vi "all_of_one.vi"() -> ()   [LabVIEW 2020]
uses:
  c112fc2c-5164-4be4-9a52-92eec6d539c9.vi
  3d77a3c8-4017-4604-99a2-a5cb9d14e92c.vi
  <vilib>/Instr/_visa.llb/VISA Configure Serial Port (Instr).vi
  <vilib>/Utility/file.llb/Read Delimited Spreadsheet (DBL).vi
panel:
  out "stop":bool
  in  "Tab Control":enum32{"Path", "GPS", "LiDAR", "ETC"}(tab)
  out "CMD_2_ERP":T1
  out "Tracking_Error(m)":dbl
  in  "A/M":bool=TRUE
  in  "Vel":dbl=4.0 format="%#_13g"
  out "Index(near vehicle)":i32
  out "Steer_CMD(Deg)":dbl
  out "XY Graph 2":T2(graph)
  out "ERP_Receive":T3
  in  "file path (dialog if empty)":path caption="RDDF"
  out "TM_X(lat)":dbl format="%-#_10g M"
  out "TM_Y(long)":dbl format="%-#_10g M"
  in  "Serial Name":refnum<visa-resource-name>="COM8"
  out "ERP_Serial_DATA(RAW)":string
  out "Brake":u8
  out "XYGraph":cluster{"array":dbl[], "array":dbl[]}[](graph)
  in  "VISA resource name":refnum<visa-resource-name>
  in  "baud rate (115200)":u32=9600
  out "True Heading":string
  out "도분초(lon)":string
  out "도(lon)":string
  out "도분초(lat)":string
  out "도(lat)":string
  out "Latitude":dbl
  out "Longtitude":dbl
  out "UTC":dbl
  out "error out":errorcluster
  out "X(N)":dbl format="%#_6f"
  out "Y(E)":dbl format="%#_6f"
  in  "Refresh":bool
  out "WP_no.":i32
  out "Satellited Used":string
  out "Fix Position":string
  out "XY Graph":cluster{dbl[], dbl[]}(graph)
  out "Mixed Signal Graph":cluster{dbl[], dbl[]}[](graph)
  out "seconds":dbl
  out "minutes":dbl
  in  "channel 15":bool
  in  "channel 14":bool
  in  "channel 13":bool
  in  "channel 12":bool
  in  "channel 11":bool
  in  "channel 10":bool
  in  "channel 9":bool=TRUE
  in  "channel 8":bool=TRUE
  in  "channel 7":bool=TRUE
  in  "channel 6":bool=TRUE
  in  "channel 5":bool
  in  "channel 4":bool
  in  "channel 3":bool
  in  "channel 2":bool
  in  "channel 1":bool
  in  "channel 0":bool
  in  "range(m)":dbl
  in  "점 개수":i32
  out "Path_Vel_arr":dbl[](array[numeric])
  out "Path_long_arr":dbl[](array[numeric])
  out "Path_lat_arr":dbl[](array[numeric])
  out "x_lat_path":dbl[](array[numeric])
  out "y_long_path":dbl[](array[numeric])
  out "vel. path":dbl[](array[numeric])
  out "Heading_T":dbl
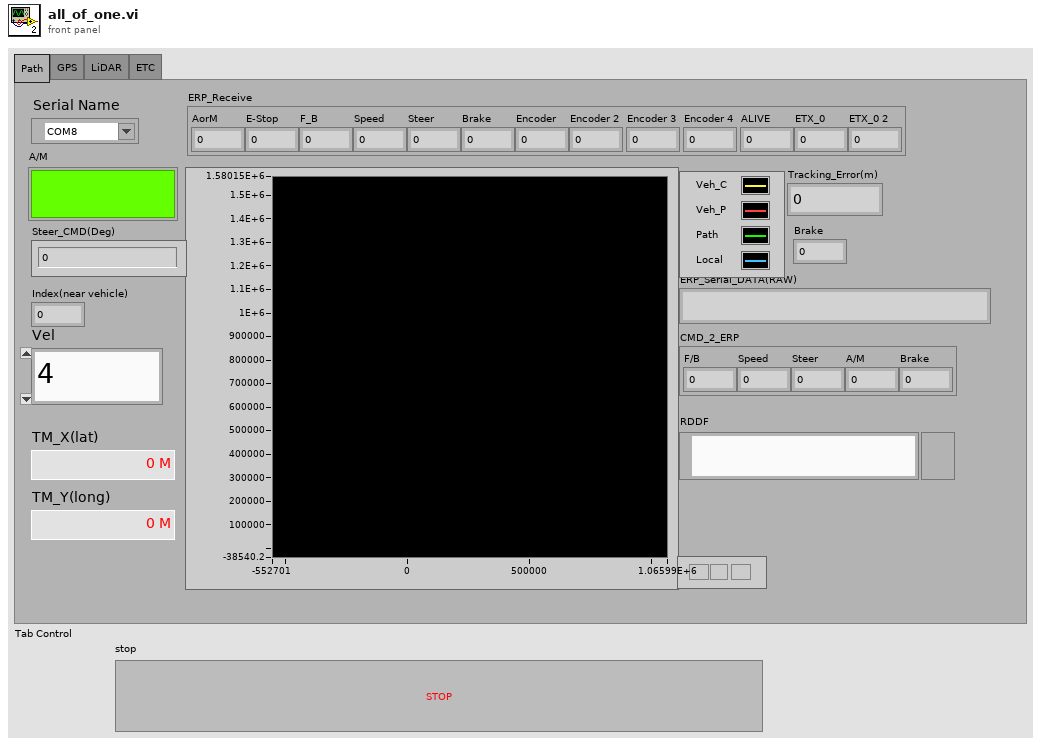
[diagram p1: front panel]
types:
  T1 = cluster{"F/B":u8, "Speed":u16, "Steer":i16, "A/M":u8, "Brake":u8}
  T2 = cluster{"y_long_path":dbl[], "x_lat_path":dbl[]}[]
  T3 = cluster{"AorM":u8, "E-Stop":u8, "F_B":u8, "Speed":u16, "Steer":i16, "Brake":u8, "Encoder":u8, "Encoder 2":u8, "Encoder 3":u8, "Encoder 4":u8, "ALIVE":u8, "ETX_0":u8, "ETX_0 2":u8}
  T4 = enum16{"open", "replace", "create", "open or create", "replace or create", "replace or create with confirmation"}
  T5 = cluster{"Path_long_arr":dbl[], "Path_lat_arr":dbl[]}
  T6 = cluster{"Path_long_arr":dbl[], "Path_lat_arr":dbl[]}[]
  T7 = cluster{"S":u8, "T":u8, "X":u8, "AorM":u8, "E-Stop":u8, "F_B":u8, "Speed":u16, "Steer":i16, "Brake":u8, "ALIVE":u8, "ETX_0":u8, "ETX_0 2":u8}
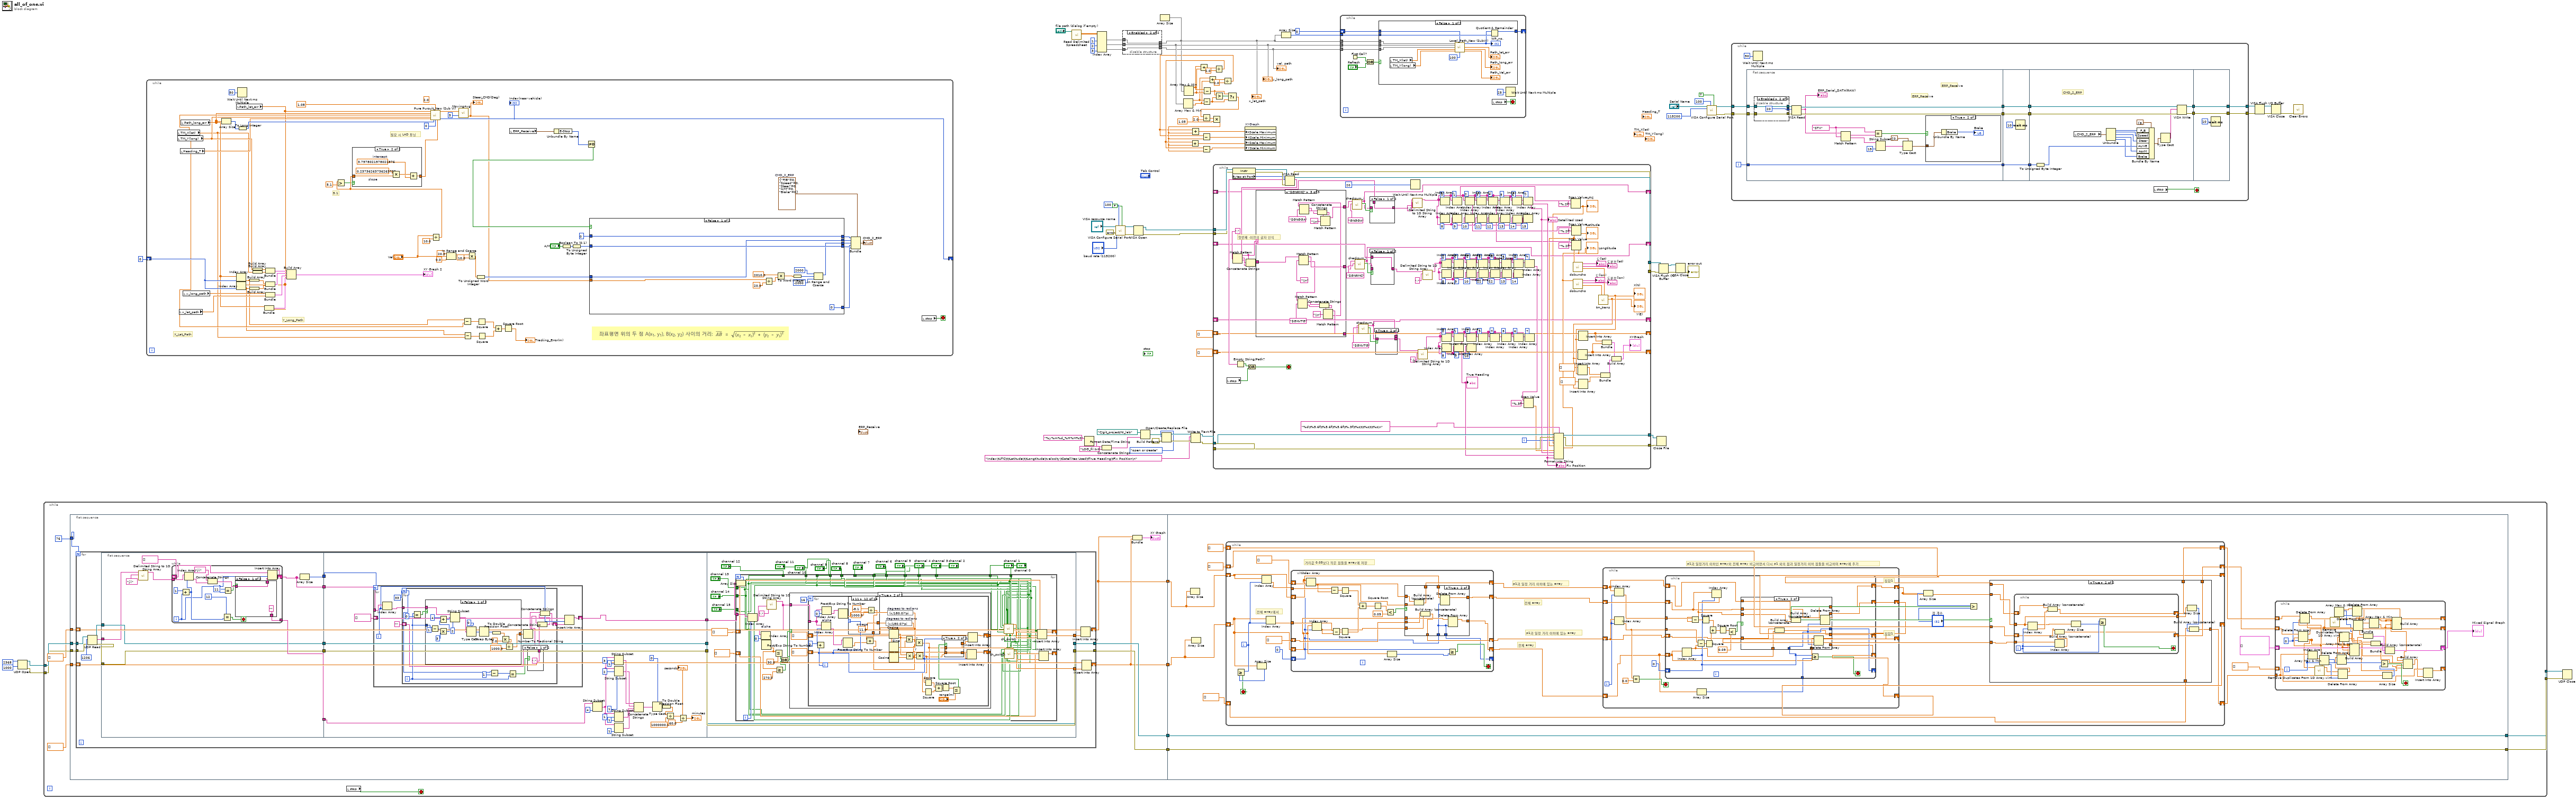
[diagram p0: block diagram]
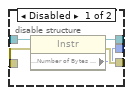
[diagram p2: hidden frame]
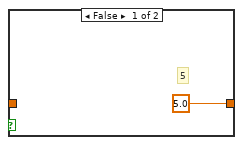
[diagram p4: hidden frame]
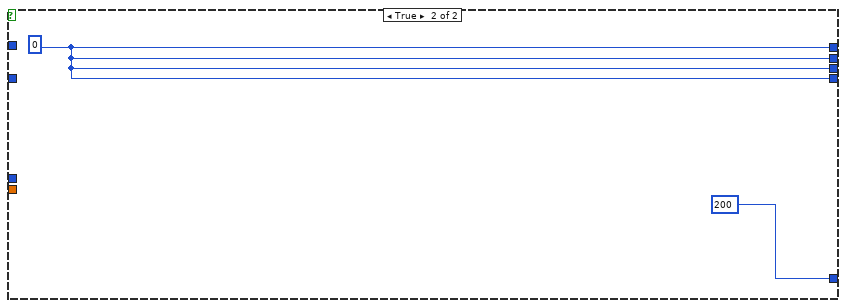
[diagram p5: hidden frame]
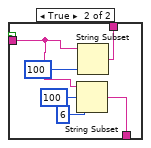
[diagram p6: hidden frame]
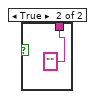
[diagram p7: hidden frame]
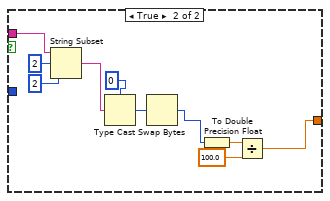
[diagram p8: hidden frame]
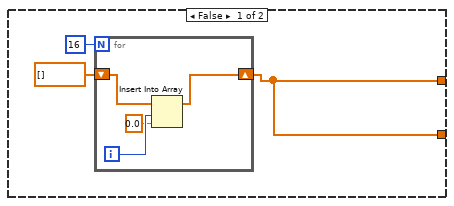
[diagram p9: hidden frame]
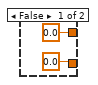
[diagram p10: hidden frame]
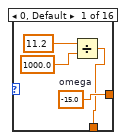
[diagram p11: hidden frame]
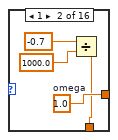
[diagram p12: hidden frame]
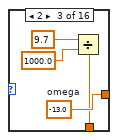
[diagram p13: hidden frame]
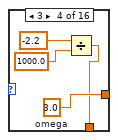
[diagram p14: hidden frame]
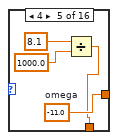
[diagram p15: hidden frame]
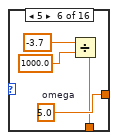
[diagram p16: hidden frame]
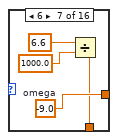
[diagram p17: hidden frame]
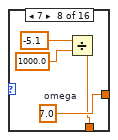
[diagram p18: hidden frame]
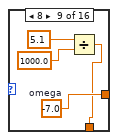
[diagram p19: hidden frame]
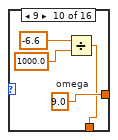
[diagram p20: hidden frame]
diagram:
  n1 = UDP Open(9:1000 ("timeout ms (25000)"), 11:u16 2368 ("port")) -> (port=w16:refnum<k16>, 0:w15:errorcluster)  [unwired: 3 in, 1 out]
  n2 = while {
    tunnel: w16 -> [w95]
    tunnel: w15 -> [w94]
    tunnel: [w91] -> w14
    tunnel: [w96] -> w13
    stop <- w85 stop-if-true
    n3 = flat-sequence {
      tunnel: w95 -> [w105]
      tunnel: w94 -> [w104]
      tunnel: dbl[] [] -> [w103]
      tunnel: dbl[] [] -> [w102]
      tunnel: 76 -> [w100]
      tunnel: [w106] -> w89
      tunnel: [w101] -> w88
      tunnel: [w98] -> w87
      tunnel: [w97] -> w86
      tunnel: [w427] -> w91
      tunnel: [w428] -> w96
      tunnel: w89 -> [w428]
      tunnel: w88 -> [w427]
      tunnel: w87 -> [w420]
      tunnel: w86 -> [w419]
      frame #0 {
        n4 = for {
          N: w100 -> [_]
          tunnel: w105 -> [w117]
          tunnel: [w119] -> w101
          tunnel: w104 -> [w116]
          tunnel: [w120] -> w106
          shift-right: [w109] -> w97
          shift-left: w103 -> [w108]
          shift-right: [w111] -> w98
          shift-left: w102 -> [w107]
          n5 = UDP Read(connection ID=w117, max size (548)=1206, 8:w116) -> (data out=w113:string, error out=w114:errorcluster, 3:w115:refnum<k16>)  [unwired: 1 in, 2 out]
          n6 = flat-sequence {
            tunnel: [w131] -> w128
            tunnel: [w130] -> w127
            tunnel: [w134] -> w126
            tunnel: [w133] -> w125
            tunnel: [w132] -> w124
            tunnel: w114 -> [w131]
            tunnel: w115 -> [w130]
            tunnel: w113 -> [w129]
            tunnel: w128 -> [w188]
            tunnel: w127 -> [w187]
            tunnel: w126 -> [w186]
            tunnel: w125 -> [w185]
            tunnel: w124 -> [w183]
            tunnel: [w188] -> w123
            tunnel: [w187] -> w122
            tunnel: [w161] -> w121
            tunnel: [w263] -> w119
            tunnel: [w264] -> w120
            tunnel: w123 -> [w264]
            tunnel: w122 -> [w263]
            tunnel: w121 -> [w261]
            tunnel: [w258] -> w110
            tunnel: [w257] -> w112
            frame #0 {
              n7 = call <vilib>:"Delimited String to 1D String Array.vi"("delimiter"="ÿî", "delimited string"=w129) -> ("string array"=w135:string[])  [unwired: 9 in]
              n8 = while {
                tunnel: w135 -> [w152]
                shift-right: [w145] -> w133
                shift-left: string[] [] -> [w144]
                tunnel: [w138] -> w132
                i -> [w141]
                stop <- w146 stop-if-true
                n9 = Add(x=1, y=w141) -> (x+y=w148:i32)
                n10 = Index Array(array=w152, index=w148) -> (element=w151:string)
                n11 = Concatenate Strings("ÿî" ("delimiter"), w151) -> (w143:string)
                n12 = Equal?(x=12, y=w148) -> (x = y?=w146:bool)
                n13 = Equal?(x=11, y=w141) -> (x = y?=w139:bool)
                n14 = case shown="False" w139 {
                  tunnel: w143 -> [w154 w156]
                  tunnel: [w154 w159] -> w142
                  tunnel: ["" w155] -> w138
                  frame False {
                  }
                  frame True {
                    n15 = String Subset(string=w156, offset (0)=100, length (rest)=6 ("length (rest)")) -> (substring=w155:string)
                    n16 = String Subset(string=w156, length (rest)=100 ("length (rest)")) -> (substring=w159:string)  [unwired: 1 in]
                  }
                }
                n17 = Insert Into Array(array=w144, index=w141, new element=w142) -> (w145:string[])
              }
              n18 = Array Size(array=w133) -> (size(s)=w134:i32)
            }
            frame #1 {
              n19 = for {
                N: w186 -> [_]
                tunnel: w185 -> [w196]
                shift-right: [w192] -> w161
                shift-left: string[] [] -> [w190]
                i -> [w193]
                n20 = Index Array(array=w196, index=w193) -> (element=w194:string)
                n21 = for {
                  N: 33 -> [w199]
                  tunnel: w194 -> [w208]
                  shift-right: [w201] -> w191
                  shift-left: "" -> [w200]
                  i -> [w207]
                  n22 = Equal?(x=w207, y=0) -> (x = y?=w209:bool)
                  n23 = case shown="False" w209 {
                    tunnel: w208 -> [w220 w238]
                    tunnel: w207 -> [w225 _]
                    tunnel: [w213 w231] -> w205
                    frame False {
                      n24 = Subtract(x=w225, y=1) -> (x-y=w226:i32)
                      n25 = Multiply(x=w226, y=3) -> (x*y=w222:i32)
                      n26 = Add(x=4 ("offset (0)"), y=w222) -> (x+y=w221:i32)
                      n27 = String Subset(string=w220, offset (0)=w221, length (rest)=2 ("length (rest)")) -> (substring=w219:string)
                      n28 = Type Cast(type=u16 0, x=w219) -> (*(type *) &x=w228:u16)
                      n29 = Swap Bytes(anything=w228) -> (byte swapped=w218:u16)
                      n30 = To Double Precision Float(number=w218) -> (double precision float=w217:dbl)
                      n31 = Multiply(x=w217, y=2.0) -> (x*y=w214:dbl)
                      n32 = Divide(x=w214, y=1000.0) -> (x/y=w213:dbl)
                    }
                    frame True {
                      n33 = String Subset(string=w238, offset (0)=2, length (rest)=2 ("length (rest)")) -> (substring=w235:string)
                      n34 = Type Cast(type=u16 0, x=w235) -> (*(type *) &x=w236:u16)
                      n35 = Swap Bytes(anything=w236) -> (byte swapped=w233:u16)
                      n36 = To Double Precision Float(number=w233) -> (double precision float=w234:dbl)
                      n37 = Divide(x=w234, y=100.0) -> (x/y=w231:dbl)
                    }
                  }
                  n38 = Subtract(x=w199, y=1) -> (x-y=w197:i32)
                  n39 = Equal?(x=w197, y=w207) -> (x = y?=w206:bool)
                  n40 = Number To Fractional String(number=w205) -> (F-format string=w204:string)  [unwired: 3 in]
                  n41 = case shown="False" w206 {
                    tunnel: ["," ""] -> w203
                    frame False {
                    }
                    frame True {
                    }
                  }
                  n42 = Concatenate Strings(w204, w203) -> (w202:string)
                  n43 = Concatenate Strings(w200, w202) -> (w201:string)
                }
                n44 = Insert Into Array(array=w190, index=w193, new element=w191) -> (w192:string[])
              }
              n45 = String Subset(string=w183, length (rest)=4 ("length (rest)")) -> (substring=w181:string)  [unwired: 1 in]
              n46 = String Subset(string=w181, offset (0)=3, length (rest)=1 ("length (rest)")) -> (substring=w173:string)
              n47 = String Subset(string=w181, offset (0)=2, length (rest)=1 ("length (rest)")) -> (substring=w172:string)
              n48 = String Subset(string=w181, offset (0)=1, length (rest)=1 ("length (rest)")) -> (substring=w171:string)
              n49 = String Subset(string=w181, length (rest)=1 ("length (rest)")) -> (substring=w170:string)  [unwired: 1 in]
              n50 = Concatenate Strings(w173, w172, w171, w170) -> (w168:string)
              n51 = Type Cast(type=u32 0, x=w168) -> (*(type *) &x=w167:u32)
              n52 = To Double Precision Float(number=w167) -> (double precision float=w166:dbl)
              n53 = Divide(x=w166, y=1000000.0) -> (x/y=w163:dbl)
              "seconds" <- w163
              n54 = Divide(x=w163, y=60.0) -> (x/y=→"minutes":dbl)
            }
            frame #2 {
              n55 = Array Size(array=w261) -> (size(s)=w262:i32)
              n56 = for {
                N: w262 -> [_]
                tunnel: w261 -> [w300]
                shift-right: [w297] -> w258
                shift-left: dbl[] [] -> [w296]
                shift-right: [w295] -> w257
                shift-left: dbl[] [] -> [w294]
                tunnel: "channel 0" -> [w289]
                tunnel: "channel 1" -> [w288]
                tunnel: "channel 2" -> [w287]
                tunnel: "channel 3" -> [w286]
                tunnel: "channel 4" -> [w285]
                tunnel: "channel 5" -> [w284]
                tunnel: "channel 6" -> [w283]
                tunnel: "channel 7" -> [w282]
                tunnel: "channel 8" -> [w281]
                tunnel: "channel 9" -> [w280]
                tunnel: "channel 10" -> [w279]
                tunnel: "channel 11" -> [w278]
                tunnel: "channel 12" -> [w277]
                tunnel: "channel 13" -> [w276]
                tunnel: "channel 14" -> [w275]
                tunnel: "channel 15" -> [w274]
                i -> [w298]
                n57 = Index Array(array=w300, index=w298) -> (element=w299:string)
                n58 = call <vilib>:"Delimited String to 1D String Array.vi"("delimiter"=",", "delimited string"=w299) -> ("string array"=w273:string[])  [unwired: 9 in]
                n59 = Index Array "alpha"(array=w273, index=0) -> (element=w271:string)
                n60 = Fract/Exp String To Number(string=w271) -> (number=w269:dbl)  [unwired: 3 in, 1 out]
                n61 = Less Or Equal?(x=w269, y=90.0 ("작거나같다")) -> (x <= y?=w267:bool)
                n62 = Greater Or Equal?(x=w269, y=270.0 ("크거나같다")) -> (x >= y?=w266:bool)
                n63 = Or(x=w267, y=w266) -> (x .or. y?=w265:bool)
                n64 = case shown="True" w265 {
                  tunnel: [w302 w311] -> w291
                  tunnel: [w302 w310] -> w290
                  tunnel: w273 -> [_ w309]
                  frame False {
                    n65 = for {
                      N: 16 -> [_]
                      shift-right: [w308] -> w302
                      shift-left: dbl[] [] -> [w305]
                      i -> [w307]
                      n66 = Insert Into Array(array=w305, index=w307, new element=0.0 ("new element/subarray")) -> (w308:dbl[])
                    }
                  }
                  frame True {
                    n67 = for {
                      N: 16 -> [_]
                      tunnel: w309 -> [w345]
                      shift-right: [w332] -> w311
                      shift-left: dbl[] [] -> [w331]
                      shift-right: [w329] -> w310
                      shift-left: dbl[] [] -> [w328]
                      i -> [w330]
                      n68 = Add(x=1, y=w330) -> (x+y=w346:i32)
                      n69 = Index Array(array=w345, index=w346) -> (element=w342:string)
                      n70 = Index Array "alpha"(array=w345, index=0) -> (element=w343:string)
                      n71 = Fract/Exp String To Number(string=w343) -> (number=w333:dbl)  [unwired: 3 in, 1 out]
                      n72 = Fract/Exp String To Number(string=w342) -> (number=w326:dbl)  [unwired: 3 in, 1 out]
                      n73 = case shown="11" w330 {
                        tunnel: [w355 w359 w363 w367 w371 w375 w379 w383 w387 w391 w395 w399 w403 w407 w411 w415] -> w341
                        tunnel: [w352 w356 w360 w364 w368 w372 w376 w380 w384 w388 w392 w396 w400 w404 w408 w412] -> w327
                        frame 0, Default {
                          w355 = -15.0  # omega
                          n74 = Divide(x=11.2, y=1000.0) -> (x/y=w352:dbl)
                        }
                        frame 1 {
                          w359 = 1.0  # omega
                          n75 = Divide(x=-0.7, y=1000.0) -> (x/y=w356:dbl)
                        }
                        frame 2 {
                          w363 = -13.0  # omega
                          n76 = Divide(x=9.7, y=1000.0) -> (x/y=w360:dbl)
                        }
                        frame 3 {
                          w367 = 3.0  # omega
                          n77 = Divide(x=-2.2, y=1000.0) -> (x/y=w364:dbl)
                        }
                        frame 4 {
                          w371 = -11.0  # omega
                          n78 = Divide(x=8.1, y=1000.0) -> (x/y=w368:dbl)
                        }
                        frame 5 {
                          w375 = 5.0  # omega
                          n79 = Divide(x=-3.7, y=1000.0) -> (x/y=w372:dbl)
                        }
                        frame 6 {
                          w379 = -9.0  # omega
                          n80 = Divide(x=6.6, y=1000.0) -> (x/y=w376:dbl)
                        }
                        frame 7 {
                          w383 = 7.0  # omega
                          n81 = Divide(x=-5.1, y=1000.0) -> (x/y=w380:dbl)
                        }
                        frame 8 {
                          w387 = -7.0  # omega
                          n82 = Divide(x=5.1, y=1000.0) -> (x/y=w384:dbl)
                        }
                        frame 9 {
                          w391 = 9.0  # omega
                          n83 = Divide(x=-6.6, y=1000.0) -> (x/y=w388:dbl)
                        }
                        frame 10 {
                          w395 = -5.0  # omega
                          n84 = Divide(x=3.7, y=1000.0) -> (x/y=w392:dbl)
                        }
                        frame 11 {
                          w399 = 11.0  # omega
                          n85 = Divide(x=-8.1, y=1000.0) -> (x/y=w396:dbl)
                        }
                        frame 12 {
                          w403 = -3.0  # omega
                          n86 = Divide(x=2.2, y=1000.0) -> (x/y=w400:dbl)
                        }
                        frame 13 {
                          w407 = 13.0  # omega
                          n87 = Divide(x=-9.7, y=1000.0) -> (x/y=w404:dbl)
                        }
                        frame 14 {
                          w411 = -1.0  # omega
                          n88 = Divide(x=0.7, y=1000.0) -> (x/y=w408:dbl)
                        }
                        frame 15 {
                          w415 = 15.0  # omega
                          n89 = Divide(x=-11.2, y=1000.0) -> (x/y=w412:dbl)
                        }
                      }
                      n90 = Add(x=w327, y=w326) -> (x+y=w325:dbl)
                      n91 = expression code="(x/180.0)*pi" "degrees to radians"(w341) -> (w340:dbl)
                      n92 = expression code="(x/180.0)*pi" "degrees to radians"(w333) -> (w339:dbl)
                      n93 = Cosine(x=w340) -> (cos(x)=w337:dbl)
                      n94 = Sine(x=w339) -> (sin(x)=w338:dbl)
                      n95 = Cosine(x=w339) -> (cos(x)=w336:dbl)
                      n96 = Multiply(x=w337, y=w338) -> (x*y=w334:dbl)
                      n97 = Multiply(x=w337, y=w336) -> (x*y=w335:dbl)
                      n98 = Multiply "x"(x=w334, y=w325) -> (x*y=w319:dbl)
                      n99 = Multiply "y"(x=w335, y=w325) -> (x*y=w317:dbl)
                      n100 = Square(x=w319) -> (x^2=w324:dbl)
                      n101 = Square(x=w317) -> (x^2=w323:dbl)
                      n102 = Add(x=w324, y=w323) -> (x+y=w322:dbl)
                      n103 = Square Root(x=w322) -> (sqrt(x)=w321:dbl)
                      n104 = Less Or Equal?(x=w321, y="range(m)") -> (x <= y?=w320:bool)
                      n105 = case shown="True" w320 {
                        tunnel: w319 -> [_ w351]
                        tunnel: [0.0 w351] -> w318
                        tunnel: w317 -> [_ w350]
                        tunnel: [0.0 w350] -> w316
                        frame False {
                        }
                        frame True {
                        }
                      }
                      n106 = Insert Into Array(array=w328, index=w330, new element=w316) -> (w329:dbl[])
                      n107 = Insert Into Array(array=w331, index=w330, new element=w318) -> (w332:dbl[])
                    }
                  }
                }
                n108 = call "ch_switch.vi"("channel 14"=w275, "channel 4"=w285, "channel 13"=w276, "channel 5"=w284, "channel 12"=w277, "channel 6"=w283, "channel 7"=w282, "channel 3"=w286, "channel 8"=w281, "channel 15"=w274, "channel 9"=w280, "channel 2"=w287, "channel 10"=w279, "channel 1"=w288, "channel 11"=w278, "channel 0"=w289, "Array in"=w291) -> ("Array out"=w292:dbl[])  [unwired: 10 in]
                n109 = call "ch_switch.vi"("channel 14"=w275, "channel 4"=w285, "channel 13"=w276, "channel 5"=w284, "channel 12"=w277, "channel 6"=w283, "channel 7"=w282, "channel 3"=w286, "channel 8"=w281, "channel 15"=w274, "channel 9"=w280, "channel 2"=w287, "channel 10"=w279, "channel 1"=w288, "channel 11"=w278, "channel 0"=w289, "Array in"=w290) -> ("Array out"=w293:dbl[])  [unwired: 10 in]
                n110 = Insert Into Array(array=w296, new element=w292) -> (w297:dbl[])  [unwired: 1 in]
                n111 = Insert Into Array(array=w294, new element=w293) -> (w295:dbl[])  [unwired: 1 in]
              }
            }
          }
          n112 = Insert Into Array(array=w108, new element=w110) -> (w109:dbl[])  [unwired: 1 in]
          n113 = Insert Into Array(array=w107, new element=w112) -> (w111:dbl[])  [unwired: 1 in]
        }
        n114 = Bundle(w97, w98) -> (→"XY Graph":cluster{dbl[], dbl[]})  [unwired: 1 in]
      }
      frame #1 {
        n115 = Array Size(array=w419) -> ()  [unwired: 1 out]
        n116 = Array Size(array=w420) -> ()  [unwired: 1 out]
        n117 = while {
          shift-right: [w471] -> _
          shift-left: w419 -> [w480]
          shift-right: [w475] -> _
          shift-left: w420 -> [w479]
          shift-right: [w472] -> w423
          shift-left: dbl[] [] -> [w474]
          shift-right: [w469] -> w422
          shift-left: dbl[] [] -> [w473]
          shift-right: [w467] -> w421
          shift-left: dbl[] [] -> [w468]
          i -> [w488]
          stop <- w489 stop-if-true
          # "전체 array에서"
          # "전체 array"
          # "p1과 일정 거리 이하에 있는 array"
          # "전체 array"
          # "p1과 일정거리 이하인 array와 전체 array 비교하면서 다시 p1 외의 점과 일정거리 이하 점들을 비교하며 array에 추가"
          # "p1과 일정 거리 이하에 있는 array"
          # "거리값 0.05보다 작은 점들을 array에 저장"
          n118 = Array Size(array=w479) -> (size(s)=w490:i32)
          n119 = Greater Or Equal?(x=w488, y=w490) -> (x >= y?=w489:bool)
          n120 = Index Array(array=w480, index=w488) -> (element=w487:dbl)
          n121 = Index Array(array=w479, index=w488) -> (element=w486:dbl)
          n122 = while {
            tunnel: w487 -> [w595]
            tunnel: w486 -> [w594]
            shift-right: [w580] -> w470
            shift-left: dbl[] [] ("array") -> [w582]
            shift-right: [w581] -> w466
            shift-left: dbl[] [] ("array") -> [w583]
            shift-right: [w577] -> w465
            shift-left: w480 -> [w579]
            shift-right: [w576] -> w464
            shift-left: w479 -> [w578]
            shift-right: [w572] -> _
            shift-left: 0 -> [w573]
            stop <- w574 stop-if-true
            n123 = Index Array(array=w579, index=w573) -> (element=w585:dbl)
            n124 = Index Array(array=w578, index=w573) -> (element=w584:dbl)
            n125 = Subtract(x=w595, y=w585) -> (x-y=w593:dbl)
            n126 = Subtract(x=w594, y=w584) -> (x-y=w592:dbl)
            n127 = Square(x=w592) -> (x^2=w590:dbl)
            n128 = Square(x=w593) -> (x^2=w591:dbl)
            n129 = Add(x=w591, y=w590) -> (x+y=w589:dbl)
            n130 = Square Root(x=w589) -> (sqrt(x)=w588:dbl)
            n131 = Less?(x=w588, y=0.09) -> (x < y?=w586:bool)
            n132 = Array Size(array=w578) -> (size(s)=w575:i32)
            n133 = case shown="True" w586 {
              tunnel: w583 -> [w602 w610]
              tunnel: w582 -> [w601 w607]
              tunnel: w585 -> [_ w609]
              tunnel: w584 -> [_ w606]
              tunnel: [w602 w608] -> w581
              tunnel: [w601 w605] -> w580
              tunnel: w579 -> [w600 w613]
              tunnel: [w600 w604] -> w577
              tunnel: w578 -> [w599 w612]
              tunnel: [w599 w611] -> w576
              tunnel: w573 -> [w597 w603]
              tunnel: [w596 w603] -> w572
              frame False {
                n134 = Add(x=1, y=w597) -> (x+y=w596:i32)
              }
              frame True {
                n135 = Build Array (concatenate)(w610, w609) -> (w608:dbl[])
                n136 = Build Array (concatenate)(w607, w606) -> (w605:dbl[])
                n137 = Delete From Array(array=w613, index=w603) -> (array with subset deleted=w604:dbl[])  [unwired: 1 in, 1 out]
                n138 = Delete From Array(array=w612, index=w603) -> (array with subset deleted=w611:dbl[])  [unwired: 1 in, 1 out]
              }
            }
            n139 = Greater Or Equal?(x=w573, y=w575) -> (x >= y?=w574:bool)
          }
          n140 = while {
            shift-right: [w521] -> w477
            shift-left: w466 -> [w524]
            shift-right: [w527] -> w476
            shift-left: w470 -> [w526]
            shift-right: [w522] -> w471
            shift-left: w465 -> [w525]
            shift-right: [w528] -> w475
            shift-left: w464 -> [w515]
            i -> [w520]
            stop <- w517 stop-if-true
            # "집합1"
            # "집합1"
            n141 = Index Array(array=w526, index=w520) -> (element=w518:dbl)
            n142 = Index Array(array=w524, index=w520) -> (element=w523:dbl)
            n143 = Equal?(x=w518, y=0.0) -> (x = y?=w517:bool)
            n144 = Array Size(array=w515) -> (size(s)=w516:i32)
            n145 = while {
              tunnel: w523 -> [w553]
              tunnel: w518 -> [w552]
              shift-right: [w540] -> _
              shift-left: 0 -> [w541]
              shift-right: [w536] -> w527
              shift-left: w526 -> [w533]
              shift-right: [w532] -> w521
              shift-left: w524 -> [w539]
              shift-right: [w531] -> w522
              shift-left: w525 -> [w535]
              shift-right: [w538] -> w528
              shift-left: w515 -> [w537]
              tunnel: w516 -> [w530]
              stop <- w542 stop-if-true
              n146 = Index Array(array=w537, index=w541) -> (element=w534:dbl)
              n147 = Subtract(x=w552, y=w534) -> (x-y=w550:dbl)
              n148 = Square(x=w550) -> (x^2=w549:dbl)
              n149 = Index Array(array=w535, index=w541) -> (element=w543:dbl)
              n150 = Subtract(x=w553, y=w543) -> (x-y=w551:dbl)
              n151 = Square(x=w551) -> (x^2=w548:dbl)
              n152 = Add(x=w548, y=w549) -> (x+y=w547:dbl)
              n153 = Square Root(x=w547) -> (sqrt(x)=w546:dbl)
              n154 = Less?(x=w546, y=0.09) -> (x < y?=w544:bool)
              n155 = case shown="True" w544 {
                tunnel: w535 -> [w554 w563]
                tunnel: w541 -> [w559 w568]
                tunnel: w543 -> [_ w571]
                tunnel: [w555 w561] -> w532
                tunnel: w533 -> [w557 w570]
                tunnel: w539 -> [w555 w564]
                tunnel: w537 -> [w560 w569]
                tunnel: [w554 w565] -> w531
                tunnel: [w560 w566] -> w538
                tunnel: [w558 w568] -> w540
                tunnel: [w557 w567] -> w536
                tunnel: w534 -> [_ w562]
                frame False {
                  n156 = Add(x=1, y=w559) -> (x+y=w558:i32)
                }
                frame True {
                  n157 = Build Array (concatenate)(w570, w562) -> (w567:dbl[])
                  n158 = Build Array (concatenate)(w564, w571) -> (w561:dbl[])
                  n159 = Delete From Array(array=w569, index=w568) -> (array with subset deleted=w566:dbl[])  [unwired: 1 in, 1 out]
                  n160 = Delete From Array(array=w563, index=w568) -> (array with subset deleted=w565:dbl[])  [unwired: 1 in, 1 out]
                }
              }
              n161 = Greater Or Equal?(x=w541, y=w530) -> (x >= y?=w542:bool)
            }
          }
          n162 = Array Size(array=w477) -> (size(s)=w482:i32)
          n163 = Greater?(x=w482, y="점 개수") -> (0:w483:bool)
          n164 = case shown="True" w483 {
            tunnel: w477 -> [_ w503]
            tunnel: w476 -> [_ w502]
            tunnel: w474 -> [w493 w501]
            tunnel: w473 -> [w492 w500]
            tunnel: [w493 w497] -> w472
            tunnel: [w492 w499] -> w469
            tunnel: w468 -> [w491 w496]
            tunnel: [w491 w495] -> w467
            frame False {
            }
            frame True {
              n165 = while {
                shift-right: [w506] -> w497
                shift-left: w501 -> [w509]
                tunnel: w503 -> [w504]
                shift-right: [w505] -> w499
                shift-left: w500 -> [w508]
                tunnel: w502 -> [w514]
                tunnel: [w504] -> w494
                i -> [w513]
                stop <- w511 stop-if-true
                n166 = Index Array(array=w504, index=w513) -> (element=w510:dbl)
                n167 = Build Array (concatenate)(w509, w510) -> (w506:dbl[])
                n168 = Index Array(array=w514, index=w513) -> (element=w507:dbl)
                n169 = Build Array (concatenate)(w508, w507) -> (w505:dbl[])
                n170 = Array Size(array=w504) -> (size(s)=w512:i32)
                n171 = Greater Or Equal?(x=w513, y=w512) -> (x >= y?=w511:bool)
              }
              n172 = Array Size(array=w494) -> (size(s)=w498:i32)
              n173 = Build Array (concatenate)(w496, w498) -> (w495:dbl[])
            }
          }
        }
        n174 = while {
          shift-right: [w458] -> _
          shift-left: w423 -> [w463]
          shift-right: [w455] -> _
          shift-left: w422 -> [w456]
          tunnel: w421 -> [w459]
          shift-right: [w453] -> w416
          shift-left: cluster{dbl[], dbl[]}[] [] -> [w452]
          shift-right: [w429] -> _
          shift-left: dbl[] [] ("array") -> [w431]
          i -> [w460]
          stop <- w461 stop-if-true
          w451 = 0 ("index")
          n175 = Index Array(array=w459, index=w460) -> (element=w457:dbl)
          n176 = Delete From Array(array=w456, length=w457, index=w451) -> (deleted portion=w442:dbl[], array with subset deleted=w455:dbl[])
          n177 = Delete From Array(array=w463, length=w457, index=w451) -> (deleted portion=w448:dbl[], array with subset deleted=w458:dbl[])
          n178 = call "Remove Duplicates From 1D Array.vim"("array"=w442) -> ("array with duplicates removed"=w440:dbl[])  [unwired: 10 in]
          n179 = Array Max & Min(array=w440) -> (max index (indices)=w438:i32, min index (indices)=w441:i32)  [unwired: 2 out]
          n180 = call "Remove Duplicates From 1D Array.vim"("array"=w448) -> ("array with duplicates removed"=w446:dbl[])  [unwired: 10 in]
          n181 = Array Max & Min(array=w446) -> (max index (indices)=w445:i32, min index (indices)=w447:i32)  [unwired: 2 out]
          n182 = Delete From Array(array=w440, index=w441) -> (array with subset deleted=w439:dbl[])  [unwired: 1 in, 1 out]
          n183 = Delete From Array(array=w439, index=w438) -> (array with subset deleted=w437:dbl[])  [unwired: 1 in, 1 out]
          n184 = Array Max & Min(array=w437) -> (max value=w433:dbl, min value=w432:dbl)  [unwired: 2 out]
          n185 = Build Array(w433, w432, w432, w433, w433) -> (w450:dbl[])
          n186 = Delete From Array(array=w446, index=w447) -> (array with subset deleted=w444:dbl[])  [unwired: 1 in, 1 out]
          n187 = Delete From Array(array=w444, index=w445) -> (array with subset deleted=w443:dbl[])  [unwired: 1 in, 1 out]
          n188 = Array Max & Min(array=w443) -> (max value=w435:dbl, min value=w434:dbl)  [unwired: 2 out]
          n189 = Bundle(w448, w442) -> (w454:cluster{dbl[], dbl[]})  [unwired: 1 in]
          n190 = Array Size(array=w459) -> (size(s)=w462:i32)
          n191 = Greater?(x=w460, y=w462) -> (0:w461:bool)
          n192 = Build Array(w435, w435, w434, w434, w435) -> (w449:dbl[])
          n193 = Bundle(w449, w450) -> (w436:cluster{dbl[], dbl[]})  [unwired: 1 in]
          n194 = Build Array (concatenate)(w452, w454, w436) -> (w453:cluster{dbl[], dbl[]}[])
          n195 = Build Array(w435, w434, w433, w432) -> (w430:dbl[])
          n196 = Insert Into Array(array=w431, new element=w430) -> (w429:dbl[])  [unwired: 1 in]
        }
        "Mixed Signal Graph" <- w416
      }
    }
    n197 = local read "stop"() -> (w85:bool)
  }
  n198 = while {
    shift-right: [w661] -> _
    shift-left: 0 -> [w658]
    stop <- w667 stop-if-true
    w633 = T1 {"F/B"=0, "Speed"=0, "Steer"=0, "A/M"=0, "Brake"=0}  # CMD_2_ERP
    (unwired) 2.0 ("L")
    # "5.1"
    # "X_Lat_Path"
    # "Y_Long_Path"
    # "필요 시 LAD 튜닝"
    n199 = local read "TM_X(lat)"() -> (w627:dbl)
    n200 = local read "TM_Y(long)"() -> (w628:dbl)
    n201 = local read "x_lat_path"() -> (w637:dbl[])
    n202 = local read "Heading_T"() -> (w654:dbl)
    n203 = local read "Path_long_arr"() -> (w630:dbl[])
    n204 = local read "y_long_path"() -> (w638:dbl[])
    n205 = Array Size(array=w630) -> (size(s)=w662:i32)
    n206 = local read "Path_lat_arr"() -> (w629:dbl[])
    n207 = Index Array(array=w630, index=w658) -> (element=w618:dbl)
    n208 = Index Array(array=w629, index=w658) -> (element=w617:dbl)
    n209 = Wait Until Next ms Multiple(millisecond multiple=u32 50 ("ms 배수")) -> ()  [unwired: 1 out]
    n210 = To Long Integer(number=w662) -> (32bit integer=w660:i32)
    n211 = Build Array(w618) -> (w669:dbl[])
    n212 = Build Array(w617) -> (w668:dbl[])
    n213 = Build Array(w628) -> (w671:dbl[])
    n214 = Build Array(w627) -> (w670:dbl[])
    n215 = Bundle("Path_long_arr"=w630, "Path_lat_arr"=w629) -> (w650:T5)  [unwired: 1 in]
    n216 = Bundle(w671, w670) -> (w656:cluster{dbl[], dbl[]})  [unwired: 1 in]
    n217 = Bundle(w669, w668) -> (w655:cluster{dbl[], dbl[]})  [unwired: 1 in]
    n218 = Bundle("y_long_path"=w638, "x_lat_path"=w637) -> (w657:cluster{"y_long_path":dbl[], "x_lat_path":dbl[]})  [unwired: 1 in]
    n219 = Build Array(w656, w655, w657, w650) -> (→"XY Graph 2":T6)
    n220 = Divide(x="Vel", y=10.0) -> (x/y=w651:dbl)
    n221 = Greater?(x=w651, y=5.1) -> (0:w616:bool)
    n222 = case shown="True" w616 {
      tunnel: w651 -> [_ w677]
      tunnel: [5.0 w676] -> w653
      frame False {
        # "5"
      }
      frame True {
        w678 = 3.7978021978021976  # intercept
        w680 = 0.23736263736263735  # slope
        n223 = Multiply(x=w680, y=w677) -> (x*y=w679:dbl)
        n224 = Add(x=w679, y=w678) -> (x+y=w676:dbl)
      }
    }
    n225 = call "Pure Pursuit_New (Sub VI).vi"("x_lat_path"=w629, "L"=1.08, "y_long_path"=w630, "X_Current"=w627, "Y_Current"=w628, "Heading_Current"=w654, "#pnt"=w660, "WP no_pre"=0, "LAD"=w653) -> ("Steer_CMD(Deg)"=w626:dbl, "Index(near vehicle)"=w661:i32)  [unwired: 5 in]
    "Index(near vehicle)" <- w661
    n226 = In Range and Coerce(upper limit=20.0 ("상위 리미트"), x="Vel", lower limit=0.0 ("하위 리미트")) -> (coerced(x)=w642:dbl)  [unwired: 1 out]
    n227 = call "MovingAvg.vi"("입력"=w626, "이동평균을 구할 자료의 개수"=u16 5) -> ("이동평균"=w614:dbl)  [unwired: 2 out]
    "Steer_CMD(Deg)" <- w614
    n228 = Subtract(x=w618, y=w628) -> (x-y=w623:dbl)
    n229 = Subtract(x=w617, y=w627) -> (x-y=w622:dbl)
    n230 = Multiply(x=w642, y=10.0) -> (x*y=w640:dbl)
    n231 = To Unsigned Word Integer(number=w640) -> (unsigned 16bit integer=w646:u16)
    n232 = Square(x=w623) -> (x^2=w621:dbl)
    n233 = Square(x=w622) -> (x^2=w620:dbl)
    n234 = Add(x=w621, y=w620) -> (x+y=w619:dbl)
    n235 = Square Root(x=w619) -> (sqrt(x)=→"Tracking_Error(m)":dbl)
    n236 = local read "ERP_Receive"() -> (w664:T3)
    n237 = Unbundle By Name(w664) -> ("E-Stop"=w665:u8)
    n238 = Boolean To (0,1)(Boolean="A/M") -> (0, 1=w649:i16)
    n239 = To Unsigned Byte Integer(number=w649) -> (unsigned 8bit integer=w631:u8)
    n240 = Not Equal To 0?(x=w665) -> (x != 0?=w645:bool)
    n241 = case shown="False" w645 {
      tunnel: u8 0 -> [w693 _]
      tunnel: [w693 w695] -> w674
      tunnel: [w690 w695] -> w673
      tunnel: [w682 w695] -> w672
      tunnel: [w692 w695] -> w648
      tunnel: w631 -> [w692 _]
      tunnel: w614 -> [w691 _]
      tunnel: w646 -> [w690 _]
      tunnel: [u8 0 u8 200] -> w634
      frame False {
        n242 = Divide(x=w691, y=20.0) -> (x/y=w688:dbl)
        n243 = Multiply(x=2010.0, y=w688) -> (x*y=w687:dbl)
        n244 = To Word Integer(number=w687) -> (16bit integer=w689:i16)
        n245 = In Range and Coerce(upper limit=i16 2000 ("상위 리미트"), x=w689, lower limit=i16 -2000 ("하위 리미트")) -> (coerced(x)=w682:i16)  [unwired: 1 out]
      }
      frame True {
        w695 = u8 0
      }
    }
    n246 = Bundle(cluster=w633, "F/B"=w674, "Speed"=w673, "Steer"=w672, "A/M"=w648, "Brake"=w634) -> (→"CMD_2_ERP":T1)
    n247 = local read "stop"() -> (w667:bool)
  }
  n248 = call-poly <vilib>:"Read Delimited Spreadsheet.vi"("file path (dialog if empty)"="file path (dialog if empty)") -> ("all rows"=w23:dbl[][])  [unwired: 9 in, 5 out]
  n249 = Format Date/Time String(time format string (%c)="%y%m%d_%H%M%S") -> (date/time string=w56:string)  [unwired: 2 in]
  n250 = Index Array(array=w23, index (col) #1=1 ("비활성화된 인덱스 (열)"), index (col) #2=2 ("인덱스 (열)"), index (col) #3=3 ("인덱스 (열)")) -> (element #1=w50:dbl[], element #2=w49:dbl[], element #3=w48:dbl[])  [unwired: 3 in]
  n251 = Concatenate Strings(w56, "LOG_fil.txt" ("string")) -> (w54:string)
  n252 = call-poly "VISA Configure Serial Port"("VISA resource name"="VISA resource name", "timeout (10sec)"=u32 100, "Enable Termination\nChar (T)"=FALSE ("Enable Termination\nChar (T)"), "baud rate (9600)"="baud rate (115200)", "error in (no error)"=errorcluster {"status"=FALSE, "code"=0, "source"=""}) -> ("VISA resource name out"=w68:refnum<visa-resource-name>, "error out"=w69:errorcluster)  [unwired: 9 in]
  n253 = disable-structure shown="Enabled" {
    disable-tunnel: w50 -> [w702 w705]
    disable-tunnel: w49 -> [w701 w704]
    disable-tunnel: w48 -> [w700 w703]
    disable-tunnel: [w699 w704] -> w27
    disable-tunnel: [w698 w703] -> w25
    disable-tunnel: [w697 w705] -> w24
    frame Disabled {
      n254 = call "InfPath(SubVI).vi"("Mod dist."=20.0, "vel."=w700, "y_long"=w701, "x_lat"=w702) -> ("vel. path"=w698:dbl[], "y_long_path"=w699:dbl[], "x_lat_path"=w697:dbl[])  [unwired: 1 out]
    }
    frame Enabled {
    }
  }
  "x_lat_path" <- w24
  "y_long_path" <- w27
  "vel. path" <- w25
  n255 = VISA Open(error in (no error)=w69, VISA resource name=w68) -> (VISA resource name=w67:refnum<visa-resource-name>, error out=w66:errorcluster)  [unwired: 3 in]
  n256 = Build Path(base path=path "C:/git_project/NI_lab", name or relative path=w54) -> (appended path=w82:path)
  n257 = Array Size(array=w24) -> ()  [unwired: 1 out]
  n258 = Open/Create/Replace File(file path (use dialog)=w82, error in=errorcluster {"status"=FALSE, "code"=0, "source"=""}, operation (0:open)=T4."open or create") -> (refnum out=w83:refnum<file>, error out=w84:errorcluster)  [unwired: 3 in, 1 out]
  n259 = Array Max & Min(array=w27) -> (max value=w36:dbl, min value=w35:dbl)  [unwired: 2 out]
  n260 = Array Max & Min(array=w24) -> (max value=w42:dbl, min value=w41:dbl)  [unwired: 2 out]
  n261 = Write to Text File(file (use dialog)=w83, text="Index\tUTC\t\tLatitude\t\tLongtitude\tvelocity\tSatellites Used\tTrue Heading\tFix Position\n", error in=w84) -> (refnum out=w75:refnum<file>, error out=w74:errorcluster)  [unwired: 1 in, 1 out]
  n262 = Add(x=w42, y=w41) -> (x+y=w39:dbl)
  n263 = Subtract(x=w36, y=w35) -> (x-y=w45:dbl)
  n264 = Subtract(x=w42, y=w41) -> (x-y=w46:dbl)
  n265 = Add(x=w36, y=w35) -> (x+y=w38:dbl)
  n266 = while {
    tunnel: w74 -> [w776]
    tunnel: [w775] -> w76
    tunnel: w75 -> [w778]
    tunnel: [w777] -> w77
    tunnel: w67 -> [w773]
    tunnel: w66 -> [w772]
    tunnel: [w761] -> w65
    tunnel: [w760] -> w64
    shift-right: [w716] -> _
    shift-left: _ -> [w740]
    shift-right: [w712] -> _
    shift-left: _ -> [w738]
    shift-right: [w709] -> _
    shift-left: _ -> [w736]
    shift-right: [w734] -> _
    shift-left: dbl[] [] -> [w735]
    shift-right: [w732] -> _
    shift-left: dbl[] [] -> [w733]
    i -> [w759]
    stop <- w826 stop-if-true
    # "첫번째 ,이전의 글자 인식"
    n267 = local read "stop"() -> (w706:bool)
    n268 = property class="Instr"(reference=w773, error in=w772) -> (reference out=w771:refnum<visa-resource-name>, error out=w770:errorcluster, "Bytes at Port"=w758:u32)
    n269 = VISA Read(VISA resource name=w771, byte count=w758, error in (no error)=w770) -> (VISA resource name out=w761:refnum<visa-resource-name>, read buffer=w753:string, error out=w760:errorcluster)  [unwired: 1 out]
    n270 = Match Pattern(string=w753, regular expression=",") -> (before substring=w750:string, match substring=w749:string, after substring=w748:string)  [unwired: 1 in, 1 out]
    n271 = Empty String/Path?(string/path=w753) -> (empty?=w827:bool)
    n272 = Concatenate Strings(w750, w749, w748) -> (w751:string)
    n273 = Or(x=w827, y=w706) -> (x .or. y?=w826:bool)
    n274 = case shown="\"$GNRMC\"" w750 {
      tunnel: w751 -> [w850 w867 w882]
      tunnel: [w849 w859 w869] -> w718
      tunnel: [w842 w852 w881] -> w714
      tunnel: [w835 w865 w875] -> w710
      frame "$GNGGA", Default {
        n275 = Match Pattern(string=w850, regular expression="\\n") -> (before substring=w849:string, after substring=w848:string)  [unwired: 1 in, 2 out]
        n276 = Match Pattern(string=w848, regular expression="$GNRMC") -> (match substring=w845:string, after substring=w844:string)  [unwired: 1 in, 2 out]
        n277 = Concatenate Strings(w845, w844) -> (w843:string)
        n278 = Match Pattern(string=w843, regular expression="\\n") -> (before substring=w842:string, after substring=w839:string)  [unwired: 1 in, 2 out]
        n279 = Match Pattern(string=w839, regular expression="$GNVTG") -> (match substring=w837:string, after substring=w836:string)  [unwired: 1 in, 2 out]
        n280 = Concatenate Strings(w837, w836) -> (w840:string)
        n281 = Match Pattern(string=w840, regular expression="\\n") -> (before substring=w835:string)  [unwired: 1 in, 3 out]
      }
      frame "$GNVTG" {
        n282 = Match Pattern(string=w867, regular expression="\\n") -> (before substring=w865:string, after substring=w864:string)  [unwired: 1 in, 2 out]
        n283 = Match Pattern(string=w864, regular expression="$GNGGA") -> (match substring=w861:string, after substring=w860:string)  [unwired: 1 in, 2 out]
        n284 = Concatenate Strings(w861, w860) -> (w862:string)
        n285 = Match Pattern(string=w862, regular expression="\\n") -> (before substring=w859:string, after substring=w858:string)  [unwired: 1 in, 2 out]
        n286 = Match Pattern(string=w858, regular expression="$GNRMC") -> (match substring=w854:string, after substring=w853:string)  [unwired: 1 in, 2 out]
        n287 = Concatenate Strings(w854, w853) -> (w855:string)
        n288 = Match Pattern(string=w855, regular expression="\\n") -> (before substring=w852:string)  [unwired: 1 in, 3 out]
      }
      frame "$GNRMC" {
        n289 = Match Pattern(string=w882, regular expression="\\n") -> (before substring=w881:string, after substring=w880:string)  [unwired: 1 in, 2 out]
        n290 = Match Pattern(string=w880, regular expression="$GNVTG") -> (match substring=w876:string, after substring=w877:string)  [unwired: 1 in, 2 out]
        n291 = Concatenate Strings(w876, w877) -> (w878:string)
        n292 = Match Pattern(string=w878, regular expression="\\n") -> (before substring=w875:string, after substring=w874:string)  [unwired: 1 in, 2 out]
        n293 = Match Pattern(string=w874, regular expression="$GNGGA") -> (match substring=w871:string, after substring=w870:string)  [unwired: 1 in, 2 out]
        n294 = Concatenate Strings(w871, w870) -> (w872:string)
        n295 = Match Pattern(string=w872, regular expression="\\n") -> (before substring=w869:string)  [unwired: 1 in, 3 out]
      }
    }
    n296 = call "checksum_i.vi"("check dataName"="GNGGA", "string"=w718) -> ("Boolean"=w717:bool, "String"=w716:string)  [unwired: 8 in]
    n297 = call "checksum_i.vi"("check dataName"="$GNRMC", "string"=w714) -> ("Boolean"=w713:bool, "String"=w712:string)  [unwired: 8 in]
    n298 = call "checksum_i.vi"("check dataName"="$GNVTG", "string"=w710) -> ("Boolean"=w708:bool, "String"=w709:string)  [unwired: 8 in]
    n299 = case shown="False" w717 {
      tunnel: [w833 w834] -> w741
      tunnel: w716 -> [_ w834]
      tunnel: w740 -> [w833 _]
      frame False {
      }
      frame True {
      }
    }
    n300 = case shown="False" w713 {
      tunnel: w712 -> [_ w832]
      tunnel: [w831 w832] -> w739
      tunnel: w738 -> [w831 _]
      frame False {
      }
      frame True {
      }
    }
    n301 = case shown="True" w708 {
      tunnel: w709 -> [_ w830]
      tunnel: [w829 w830] -> w737
      tunnel: w736 -> [w829 _]
      frame False {
      }
      frame True {
      }
    }
    n302 = Wait Until Next ms Multiple(millisecond multiple=u32 20) -> ()  [unwired: 1 out]
    n303 = call <vilib>:"Delimited String to 1D String Array.vi"("delimiter"=",", "delimited string"=w741) -> ("string array"=w825:string[])  [unwired: 9 in]
    n304 = call <vilib>:"Delimited String to 1D String Array.vi"("delimiter"=",", "delimited string"=w737) -> ("string array"=w790:string[])  [unwired: 9 in]
    n305 = call <vilib>:"Delimited String to 1D String Array.vi"("delimiter"=",", "delimited string"=w739) -> ("string array"=w807:string[])  [unwired: 9 in]
    n306 = Index Array(array=w825, index=0) -> ()  [unwired: 1 out]
    n307 = Index Array(array=w825, index=8) -> ()  [unwired: 1 out]
    n308 = Index Array(array=w807, index=0) -> ()  [unwired: 1 out]
    n309 = Index Array(array=w790, index=0) -> ()  [unwired: 1 out]
    n310 = Index Array(array=w807, index=8) -> ()  [unwired: 1 out]
    n311 = Index Array(array=w790, index=8) -> ()  [unwired: 1 out]
    n312 = Index Array(array=w825, index=1) -> (element=w766:string)
    n313 = Index Array(array=w825, index=9) -> ()  [unwired: 1 out]
    n314 = Index Array(array=w807, index=1) -> ()  [unwired: 1 out]
    n315 = Index Array(array=w807, index=9) -> ()  [unwired: 1 out]
    n316 = Index Array(array=w790, index=1) -> (element=w769:string)
    "True Heading" <- w769
    n317 = Index Array(array=w790, index=9) -> ()  [unwired: 1 out]
    n318 = Index Array(array=w825, index=2) -> (element=w763:string)
    n319 = Index Array(array=w825, index=10) -> ()  [unwired: 1 out]
    n320 = Index Array(array=w807, index=2) -> ()  [unwired: 1 out]
    n321 = Index Array(array=w807, index=10) -> ()  [unwired: 1 out]
    n322 = Index Array(array=w790, index=2) -> ()  [unwired: 1 out]
    n323 = Index Array(array=w790, index=10) -> ()  [unwired: 1 out]
    n324 = Index Array(array=w825, index=3) -> ()  [unwired: 1 out]
    n325 = Index Array(array=w825, index=11) -> ()  [unwired: 1 out]
    n326 = Index Array(array=w807, index=3) -> ()  [unwired: 1 out]
    n327 = Index Array(array=w790, index=3) -> ()  [unwired: 1 out]
    n328 = Index Array(array=w807, index=11) -> ()  [unwired: 1 out]
    n329 = Index Array(array=w825, index=4) -> (element=w762:string)
    n330 = Index Array(array=w825, index=12) -> ()  [unwired: 1 out]
    n331 = Index Array(array=w807, index=4) -> ()  [unwired: 1 out]
    n332 = Index Array(array=w790, index=4) -> ()  [unwired: 1 out]
    n333 = Index Array(array=w807, index=12) -> ()  [unwired: 1 out]
    n334 = Index Array(array=w825, index=5) -> ()  [unwired: 1 out]
    n335 = Index Array(array=w825, index=13) -> ()  [unwired: 1 out]
    n336 = Index Array(array=w807, index=5) -> ()  [unwired: 1 out]
    n337 = Index Array(array=w790, index=5) -> ()  [unwired: 1 out]
    n338 = Index Array(array=w807, index=13) -> ()  [unwired: 1 out]
    n339 = Index Array(array=w825, index=6) -> (element=w768:string)
    "Fix Position" <- w768
    n340 = Index Array(array=w825, index=14) -> ()  [unwired: 1 out]
    n341 = Index Array(array=w807, index=6) -> ()  [unwired: 1 out]
    n342 = Index Array(array=w790, index=6) -> ()  [unwired: 1 out]
    n343 = Index Array(array=w807, index=14) -> ()  [unwired: 1 out]
    n344 = Index Array(array=w825, index=7) -> (element=w767:string)
    "Satellited Used" <- w767
    n345 = Index Array(array=w825, index=15) -> ()  [unwired: 1 out]
    n346 = Index Array(array=w807, index=7) -> (element=w722:string)
    n347 = Scan Value(string=w722, format string="%.3f") -> (value=w721:dbl)  [unwired: 1 in, 1 out]
    n348 = Index Array(array=w790, index=7) -> ()  [unwired: 1 out]
    n349 = Scan Value(string=w766, format string="%.2f") -> (value=w707:dbl)  [unwired: 1 in, 1 out]
    "UTC" <- w707
    n350 = Scan Value(string=w763, format string="%.2f") -> (value=w746:dbl)  [unwired: 1 in, 1 out]
    "Latitude" <- w746
    n351 = Scan Value(string=w762, format string="%.2f") -> (value=w745:dbl)  [unwired: 1 in, 1 out]
    "Longtitude" <- w745
    n352 = Format Into String(format string="%d\t%5.6f\t%5.6f\t%5.6f\t%.3f\t%s\t\t%s\t\t%s\n", initial string=w778, error in=w776, w759, w707, w746, w745, w721, w767, w769, w768) -> (resulting string=w777:refnum<file>, error out=w775:errorcluster)
    n353 = call "dobuncho.vi"("Numeric in"=w746) -> ("Numeric out"=w747:dbl, "String"=→"도분초(lat)":string, "String 2"=→"도(lat)":string)  [unwired: 8 in]
    n354 = call "dobuncho.vi"("Numeric in"=w745) -> ("Numeric out"=w742:dbl, "String"=→"도분초(lon)":string, "String 2"=→"도(lon)":string)  [unwired: 8 in]
    n355 = call "tm_trans.vi"("Long"=w742, "Lat"=w747) -> ("Numeric"=w730:dbl, "out_pt"=w731:dbl)  [unwired: 8 in]
    "Y(E)" <- w730
    "X(N)" <- w731
    n356 = Insert Into Array(array=w733, new element=w730) -> (w732:dbl[])  [unwired: 1 in]
    n357 = Insert Into Array(array=dbl[] [], new element=w731) -> (w727:dbl[])  [unwired: 1 in]
    n358 = Insert Into Array(array=dbl[] [], new element=w730) -> (w726:dbl[])  [unwired: 1 in]
    n359 = Insert Into Array(array=w735, new element=w731) -> (w734:dbl[])  [unwired: 1 in]
    n360 = Bundle("array"=w727, "array"=w726) -> (w725:cluster{"array":dbl[], "array":dbl[]})  [unwired: 1 in]
    n361 = Bundle(w734, w732) -> (w724:cluster{dbl[], dbl[]})  [unwired: 1 in]
    n362 = Build Array(w724, w725) -> (→"XYGraph":cluster{"array":dbl[], "array":dbl[]}[])
  }
  n363 = Divide(x=w39, y=2.0) -> (x/y=w33:dbl)
  n364 = Greater?(x=w46, y=w45) -> (0:w47:bool)
  n365 = Divide(x=w38, y=2.0) -> (x/y=w21:dbl)
  n366 = Select(t=w46, s=w47, f=w45) -> (s? t:f=w43:dbl)
  n367 = Divide(x=w43, y=2.0) -> (x/y=w34:dbl)
  n368 = Multiply(x=w34, y=1.05) -> (x*y=w32:dbl)
  n369 = Add(x=w33, y=w32) -> (x+y=w30:dbl)
  n370 = Add(x=w21, y=w32) -> (x+y=w28:dbl)
  n371 = Subtract(x=w21, y=w32) -> (x-y=w29:dbl)
  n372 = Subtract(x=w33, y=w32) -> (x-y=w31:dbl)
  n373 = property on="XYGraph" class="XYGraph (strict)"("XScale.Maximum"=w28, "XScale.Minimum"=w29, "YScale.Maximum"=w30, "YScale.Minimum"=w31) -> ()  [unwired: 2 in, 2 out]
  n374 = Array Size(array=w24) -> (size(s)=w26:i32)
  n375 = while {
    tunnel: w24 -> [w895]
    tunnel: w27 -> [w894]
    tunnel: w25 -> [w892]
    tunnel: w26 -> [w891]
    shift-right: [w890] -> _
    shift-left: 0 ("Index0") -> [w893]
    stop <- w896 stop-if-true
    n376 = First Call?() -> (First Call?: T/F=w888:bool)
    n377 = Or(x=w888, y="Refresh") -> (x .or. y?=w889:bool)
    n378 = case shown="False" w889 {
      tunnel: w895 -> [w897 w916]
      tunnel: w894 -> [w899 w915]
      tunnel: w893 -> [w904 _]
      tunnel: w892 -> [w898 _]
      tunnel: w891 -> [w908 _]
      tunnel: [w909 w910] -> w890
      frame False {
        n379 = local read "TM_X(lat)"() -> (w907:dbl)
        n380 = local read "TM_Y(long)"() -> (w906:dbl)
        n381 = call "Local_Path_New (SubVI).vi"("x_lat_arr"=w897, "WP no_pre"=w904, "y_long_arr"=w899, "vel_arr"=w898, "x_lat_c"=w907, "y_long_c"=w906, "# of pnt"=100) -> ("INDEX(Near Point)"=w900:i32, "Lat(Local)"=→"Path_lat_arr":dbl[], "Long(Local)"=→"Path_long_arr":dbl[], "Vel(Local)"=→"Path_Vel_arr":dbl[])  [unwired: 5 in]
        "WP_no." <- w900
        n382 = Quotient & Remainder(x=w900, y=w908) -> (x-y*floor(x/y)=w909:i32)  [unwired: 1 out]
      }
      frame True {
        n383 = local read "TM_X(lat)"() -> (w914:dbl)
        n384 = local read "TM_Y(long)"() -> (w913:dbl)
        n385 = local read "Heading_T"() -> (w912:dbl)
        n386 = call "Local_Path_Second (SubVI).vi"("heading_deg"=w912, "heading_limit"=179.0, "y_long"=w913, "x_lat"=w914, "Y_long_path"=w915, "X_lat_path"=w916) -> ("Index(near vehicle)"=w910:i32)  [unwired: 1 out]
      }
    }
    n387 = local read "stop"() -> (w896:bool)
    n388 = Wait Until Next ms Multiple(millisecond multiple=u32 25) -> ()  [unwired: 1 out]
  }
  n389 = Close File(refnum=w77, error in=w76) -> ()  [unwired: 2 out]
  n390 = VISA Flush I/O Buffer(VISA resource name=w65, error in (no error)=w64) -> (VISA resource name out=w62:refnum<visa-resource-name>, error out=w63:errorcluster)  [unwired: 1 in]
  n391 = VISA Close(VISA resource name=w62, error in (no error)=w63) -> (error out=→"error out":errorcluster)
  n392 = call-poly "VISA Configure Serial Port"("VISA resource name"="Serial Name", "timeout (10sec)"=u32 100, "Enable Termination\nChar (T)"=TRUE ("Enable Termination\nChar (T)"), "baud rate (9600)"=u32 115200) -> ("VISA resource name out"=w4:refnum<visa-resource-name>, "error out"=w3:errorcluster)  [unwired: 10 in]
  n393 = while {
    tunnel: w4 -> [w930]
    tunnel: w3 -> [w929]
    tunnel: [w927] -> w1
    tunnel: [w926] -> w5
    i -> [w928]
    stop <- w919 stop-if-true
    n394 = flat-sequence {
      tunnel: w930 -> [w948]
      tunnel: w929 -> [w947]
      tunnel: [w946] -> w925
      tunnel: [w945] -> w923
      tunnel: w928 -> [w944]
      tunnel: [w944] -> w921
      tunnel: w925 -> [w962]
      tunnel: [w962] -> w924
      tunnel: w923 -> [w961]
      tunnel: [w961] -> w922
      tunnel: w921 -> [w960]
      tunnel: [w960] -> w920
      tunnel: w924 -> [w975]
      tunnel: w922 -> [w974]
      tunnel: w920 -> [w972]
      tunnel: [w971] -> w918
      tunnel: [w970] -> w917
      tunnel: [w979] -> w926
      tunnel: [w980] -> w927
      tunnel: w918 -> [w980]
      tunnel: w917 -> [w979]
      frame #0 {
        w938 = "STX" ("검색 문자열/문자 (-)")
        # "ERP_Receive"
        # "ERP_Receive"
        n395 = disable-structure shown="Enabled" {
          disable-tunnel: w948 -> [w953 w955]
          disable-tunnel: w947 -> [w952 w956]
          disable-tunnel: [w951 w956] -> w943
          disable-tunnel: [w950 u32 20 ("timeout (10sec)")] -> w942
          disable-tunnel: [w949 w955] -> w941
          frame Disabled {
            n396 = property class="Instr"(reference=w953, error in=w952) -> (reference out=w949:refnum<visa-resource-name>, error out=w951:errorcluster, "Serial Settings:Number of Bytes at Serial Port"=w950:u32)
          }
          frame Enabled {
          }
        }
        n397 = VISA Read(VISA resource name=w941, byte count=w942, error in (no error)=w943) -> (VISA resource name out=w946:refnum<visa-resource-name>, read buffer=w936:string, error out=w945:errorcluster)  [unwired: 1 out]
        "ERP_Serial_DATA(RAW)" <- w936
        n398 = Match Pattern(string=w936, regular expression=w938) -> (match substring=w937:string, after substring=w940:string)  [unwired: 1 in, 2 out]
        n399 = Equal?(x=w938, y=w937) -> (x = y?=w935:bool)
        n400 = String Subset(string=w940, length (rest)=15 ("길이(나머지)")) -> (substring=w934:string)  [unwired: 1 in]
        n401 = Type Cast(type=T3 {"AorM"=0, "E-Stop"=0, "F_B"=0, "Speed"=0, "Steer"=0, "Brake"=0, "Encoder"=0, "Encoder 2"=0, "Encoder 3"=0, "Encoder 4"=0, "ALIVE"=0, "ETX_0"=13, "ETX_0 2"=10}, x=w934) -> (*(type *) &x=w933:T3)
        n402 = case shown="True" w935 {
          tunnel: w933 -> [_ w958]
          frame False {
          }
          frame True {
            n403 = Unbundle By Name(w958) -> ("Brake"=→"Brake":u8)
          }
        }
      }
      frame #1 {
        n404 = Wait (ms)(milliseconds to wait=u32 10 ("대기 시간(ms)")) -> ()  [unwired: 1 out]
      }
      frame #2 {
        # "CMD_2_ERP"
        n405 = To Unsigned Byte Integer(number=w972) -> (unsigned 8bit integer=w977:u8)
        n406 = local read "CMD_2_ERP"() -> (w964:T1)
        n407 = Unbundle(w964) -> ("F/B"=w969:u8, "Speed"=w968:u16, "Steer"=w967:i16, "A/M"=w965:u8, "Brake"=w963:u8)
        n408 = Bundle By Name(cluster=T7 {"S"=83, "T"=84, "X"=88, "AorM"=0, "E-Stop"=0, "F_B"=0, "Speed"=0, "Steer"=0, "Brake"=0, "ALIVE"=0, "ETX_0"=13, "ETX_0 2"=10}, "F_B"=w969, "Speed"=w968, "Steer"=w967, "ALIVE"=w977, "AorM"=w965, "Brake"=w963) -> (w976:T7)
        n409 = Type Cast(x=w976) -> (*(type *) &x=w973:string)  [unwired: 1 in]
        n410 = VISA Write(VISA resource name=w975, write buffer=w973, error in (no error)=w974) -> (VISA resource name out=w971:refnum<visa-resource-name>, error out=w970:errorcluster)  [unwired: 1 out]
      }
      frame #3 {
        n411 = Wait (ms)(milliseconds to wait=u32 10 ("대기 시간(ms)")) -> ()  [unwired: 1 out]
      }
    }
    n412 = Wait Until Next ms Multiple(millisecond multiple=u32 50 ("ms 배수")) -> ()  [unwired: 1 out]
    n413 = local read "stop"() -> (w919:bool)
  }
  n414 = VISA Flush I/O Buffer(VISA resource name=w1, error in (no error)=w5) -> (VISA resource name out=w6:refnum<visa-resource-name>, error out=w7:errorcluster)  [unwired: 1 in]
  n415 = VISA Close(VISA resource name=w6, error in (no error)=w7) -> (error out=w2:errorcluster)
  n416 = call <vilib>:"Clear Errors.vi"("error in (no error)"=w2) -> ()  [unwired: 5 in, 2 out]
  n417 = UDP Close(connection ID=w14, 8:w13) -> ()  [unwired: 2 out]
